vi "ExTestIsAvails.vi"() -> ()   [LabVIEW 2010]
panel:
  in  "stop":bool
  in  "Speed Table Index":u32
  in  "Param ID":u32
  out "Description":string
  out "Number of Enums":u32
  out "Bit Used Flag":u32 format="%.0x"
  out "Access Type":u32
  out "Data Type":u32
  out "Increment":dbl format="%.2f"
  out "Max Value":dbl format="%.2f"
  out "Min Value":dbl format="%.2f"
  out "Default Value":dbl format="%.2f"
  out "Current Value":dbl format="%.2f"
  out "Avail Flag":u8
  out "Param ID":u32
  out "error out":errorcluster
  in  "error in (no error)":errorcluster
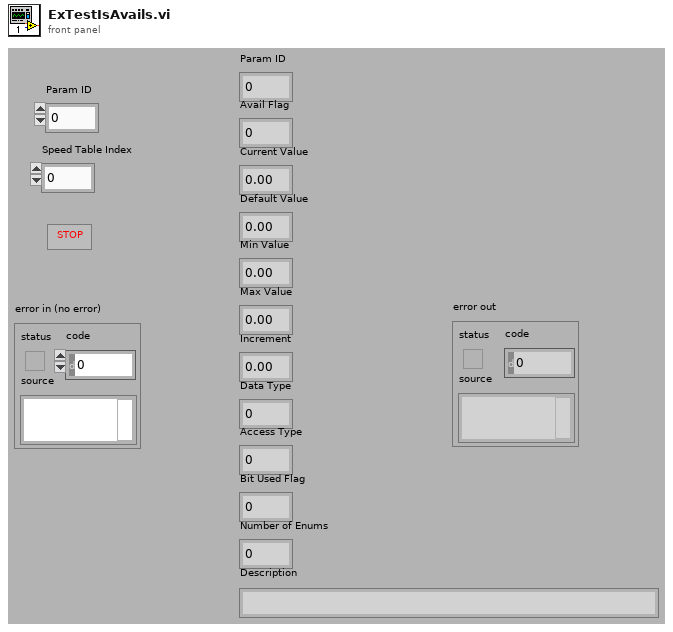
[diagram p1: front panel]
types:
  T1 = cluster{"Param ID":u32, "Avail Flag":u8, "Current Value":dbl, "Default Value":dbl, "Min Value":dbl, "Max Value":dbl, "Increment":dbl, "Data Type":u32, "Access Type":u32, "Bit Used Flag":u32, "Number of Enums":u32, "Description":string}
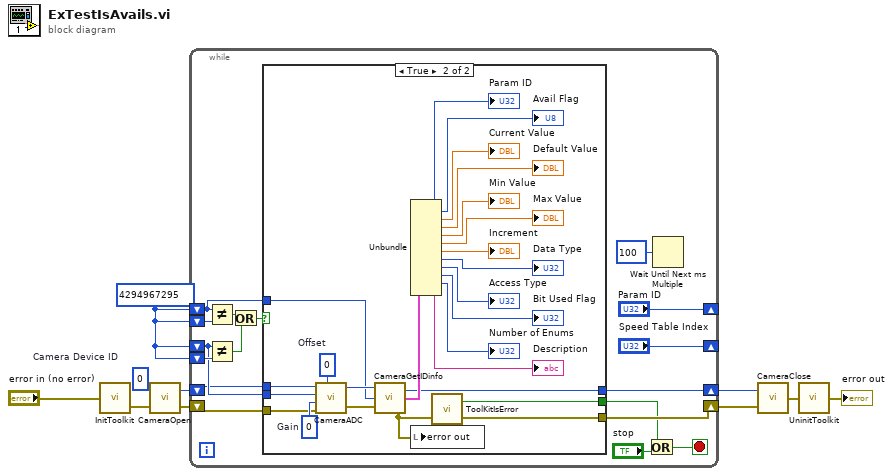
[diagram p0: block diagram]
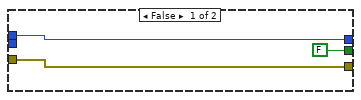
[diagram p2: hidden frame]
diagram:
  w5 = u32 4294967295
  w7 = u32 0  # Camera Device ID
  n1 = call <userlib>:"InitToolkit.vi"("error in"="error in (no error)") -> ("error out"=w6:errorcluster)
  n2 = call <userlib>:"CameraOpen.vi"("error in"=w6, "Camera Device ID"=w7) -> ("error out"=w4:errorcluster, "Camera Handle"=w3:u32)
  n3 = while {
    shift-right: ["Param ID"] -> _
    shift-left: w5 -> [w20]
    shift-right: ["Speed Table Index"] -> _
    shift-left: w5 -> [w17]
    shift-left: w5 -> [w27]
    shift-left: w5 -> [w26]
    shift-right: [w18] -> w2
    shift-left: w3 -> [w16]
    shift-right: [w13] -> w1
    shift-left: w4 -> [w19]
    stop <- w11 stop-if-true
    n4 = Not Equal?(x=w20, y=w27) -> (x != y?=w25:bool)
    n5 = Not Equal?(x=w17, y=w26) -> (x != y?=w24:bool)
    n6 = Or(x=w25, y=w24) -> (x .or. y?=w23:bool)
    n7 = case shown="True" w23 {
      tunnel: w19 -> [w29 w40]
      tunnel: w16 -> [w30 w39]
      tunnel: w20 -> [_ w36]
      tunnel: w17 -> [_ w35]
      tunnel: [w30 w34] -> w18
      tunnel: [w29 w32] -> w13
      tunnel: [FALSE ("Error Flag") w33] -> w12
      frame False {
      }
      frame True {
        w41 = u32 0  # Offset
        w42 = u32 0  # Gain
        n8 = call <userlib>:"CameraADC.vi"("Camera Handle"=w39, "Speed"=w35, "Gain"=w42, "error in (no error)"=w40, "Offset"=w41) -> ("Camera Handle"=w37:u32, "error out"=w38:errorcluster)
        n9 = call <userlib>:"CameraGetIDinfo.vi"("error in"=w38, "Param ID"=w36, "Camera handle"=w37) -> ("error out"=w31:errorcluster, "Param ID Information"=w55:T1, "Camera handle"=w34:u32)
        n10 = Unbundle(w55) -> ("Param ID"=→"Param ID":u32, "Avail Flag"=→"Avail Flag":u8, "Current Value"=→"Current Value":dbl, "Default Value"=→"Default Value":dbl, "Min Value"=→"Min Value":dbl, "Max Value"=→"Max Value":dbl, "Increment"=→"Increment":dbl, "Data Type"=→"Data Type":u32, "Access Type"=→"Access Type":u32, "Bit Used Flag"=→"Bit Used Flag":u32, "Number of Enums"=→"Number of Enums":u32, "Description"=→"Description":string)
        n11 = local write "error out"(w31) -> ()
        n12 = call <userlib>:"ToolKitIsError.vi"("error in"=w31) -> ("error out"=w32:errorcluster, "Error Flag"=w33:bool)  [unwired: 1 in]
      }
    }
    n13 = Or(x=w12, y="stop") -> (x .or. y?=w11:bool)
    n14 = Wait Until Next ms Multiple(millisecond multiple=u32 100) -> ()  [unwired: 1 out]
  }
  n15 = call <userlib>:"CameraClose.vi"("error in"=w1, "Camera Handle"=w2) -> ("error out"=w10:errorcluster)
  n16 = call <userlib>:"UninitToolkit.vi"("error in"=w10) -> ("error out"=→"error out":errorcluster)
